vi "配置.vi"() -> (2 "启用参数":T1, 3 "串口输出":refnum<visa-resource-name>)   [LabVIEW 2016, in "国弘多参数.lvlib"]
uses:
  <vilib>/Utility/miscctls.llb/LVPointTypeDef.ctl
panel:
  in  "叶绿素a启用":bool
  in  "Temp":bool
  in  "Cond":bool
  in  "Turb":bool
  in  "DO":bool
  in  "pH":bool
  in  "关闭":bool
  in  "VISA资源名称":refnum<visa-resource-name>
  # "请设置串口参数"
  # "请选择要启用的参数"
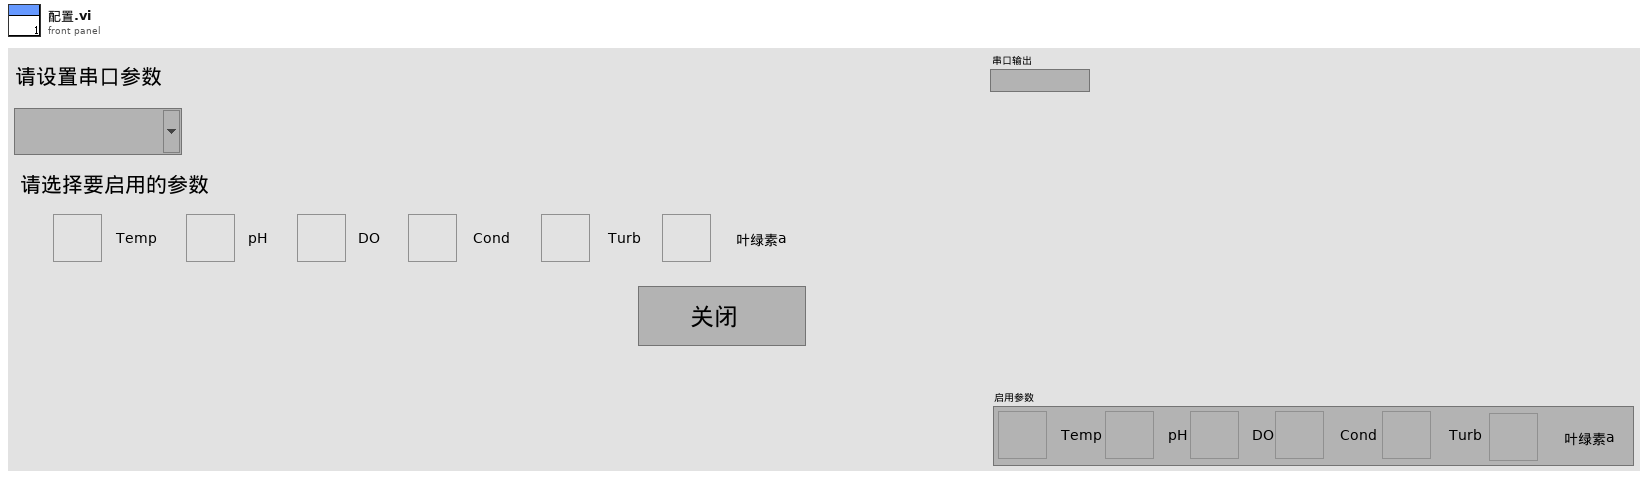
[diagram p1: front panel]
types:
  T1 = cluster{"Temp":bool, "pH":bool, "DO":bool, "Cond":bool, "Turb":bool, "叶绿素a启用":bool}
  T2 = typedef "LVPointTypeDef.ctl" = cluster{"Horizontal":i16, "Vertical":i16}
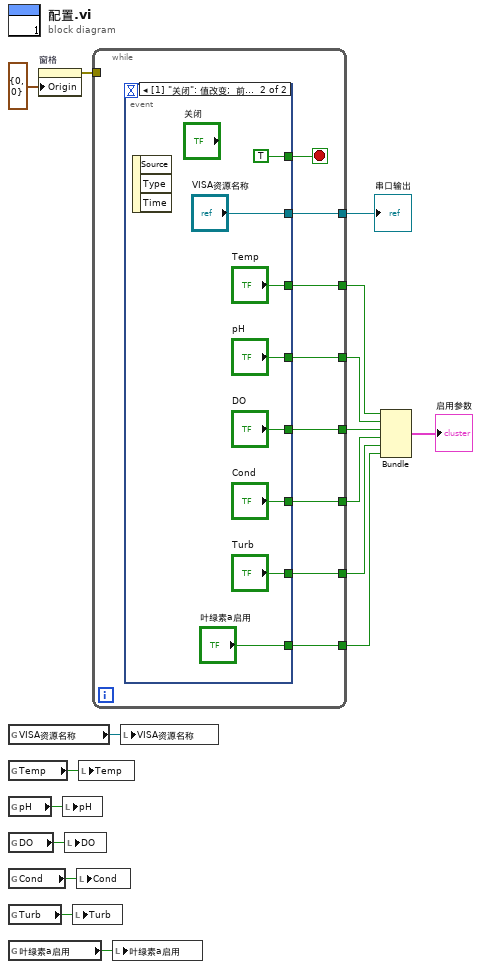
[diagram p0: block diagram]
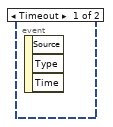
[diagram p2: hidden frame]
diagram:
  n1 = global read "断电保存变量.vi" "VISA资源名称"() -> (w10:refnum<visa-resource-name>)
  n2 = global read "断电保存变量.vi" "Temp"() -> (w5:bool)
  n3 = global read "断电保存变量.vi" "pH"() -> (w6:bool)
  n4 = global read "断电保存变量.vi" "DO"() -> (w7:bool)
  n5 = global read "断电保存变量.vi" "Cond"() -> (w8:bool)
  n6 = global read "断电保存变量.vi" "Turb"() -> (w9:bool)
  n7 = global read "断电保存变量.vi" "叶绿素a启用"() -> (w1:bool)
  n8 = property on="窗格" class="Pane"("Origin"=T2 {"Horizontal"=0, "Vertical"=0} ("原点")) -> (error out=w3:errorcluster)  [unwired: 2 in, 1 out]
  n9 = local write "pH"(w6) -> ()
  n10 = local write "DO"(w7) -> ()
  n11 = local write "Turb"(w9) -> ()
  n12 = local write "Cond"(w8) -> ()
  n13 = local write "Temp"(w5) -> ()
  n14 = while {
    tunnel: [w24] -> w17
    tunnel: [w23] -> w16
    tunnel: [w22] -> w15
    tunnel: [w21] -> w14
    tunnel: [w20] -> w13
    tunnel: [w19] -> w12
    tunnel: [w18] -> w4
    tunnel: w3 -> [_]
    stop <- w25 stop-if-true
    n15 = event shown="[1] \"关闭\": 值改变;  前面板关闭" {
      selector: _ -> [_ _]
      dyn-events: _ -> [_ _]
      timeout: _ -> [_ _]
      tunnel: [_ TRUE] -> w25
      tunnel: [_ "VISA资源名称"] -> w24
      tunnel: [_ "Temp"] -> w23
      tunnel: [_ "pH"] -> w22
      tunnel: [_ "DO"] -> w21
      tunnel: [_ "Cond"] -> w20
      tunnel: [_ "Turb"] -> w19
      tunnel: [_ "叶绿素a启用"] -> w18
      event Timeout {
        n16 = event-data() -> ()  [unwired: 1 in, 3 out]
      }
      event "关闭": Value Change; Panel Close {
        n17 = event-data() -> ()  [unwired: 1 in, 3 out]
      }
    }
  }
  "串口输出" <- w17
  n18 = local write "叶绿素a启用"(w1) -> ()
  n19 = local write "VISA资源名称"(w10) -> ()
  n20 = Bundle("Temp"=w16, "pH"=w15, "DO"=w14, "Cond"=w13, "Turb"=w12, "叶绿素a启用"=w4) -> (→"启用参数":T1)  [unwired: 1 in]
